vi "StirSticks.vi"(11 "RelayValue":T1) -> ()   [LabVIEW 2016]
uses:
  <vilib>/Rock Robotics/WPI/Relay/WPI_RelayValue.ctl
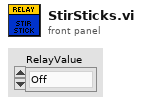
[diagram p1: front panel]
types:
  T1 = typedef "WPI_RelayValue.ctl" = enum16{"Off", "On", "Forward", "Reverse"}
  T2 = typedef "WPI_RelayDevRef.ctl" = cluster{"DevStatus":errorcluster, "Relay Channel":T3, "Relay Direction":T4}
  T3 = typedef "FPGA_DIORelayChannel.ctl" = enum8{"Relay 0", "Relay 1", "Relay 2", "Relay 3", "Invalid"}
  T4 = typedef "WPI_RelayDirection.ctl" = enum16{"Both directions", "Forward only", "Reverse only"}
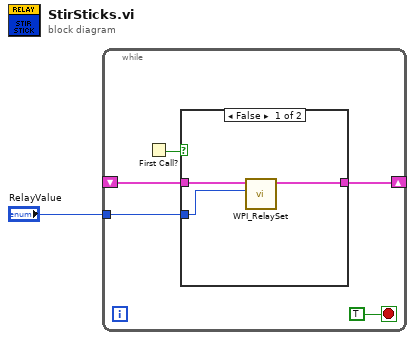
[diagram p0: block diagram]
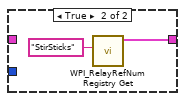
[diagram p2: hidden frame]
diagram:
  n1 = while {
    shift-right: [w4] -> _
    shift-left: _ -> [w3]
    tunnel: "RelayValue" -> [w2]
    stop <- TRUE stop-if-true
    n2 = First Call?() -> (First Call?: T/F=w5:bool)
    n3 = case shown="False" w5 {
      tunnel: [w8 w10] -> w4
      tunnel: w3 -> [w9 _]
      tunnel: w2 -> [w7 _]
      frame False {
        n4 = call <vilib>:"WPI_RelaySet.vi"("RelayValue"=w7, "RelayDevRef"=w9) -> ("RelayDevRef"=w8:T2)  [unwired: 8 in, 1 out]
      }
      frame True {
        n5 = call <vilib>:"WPI_RelayRefNum Registry Get.vi"("refnum name"="StirSticks") -> ("RelayDevRef"=w10:T2)  [unwired: 9 in, 1 out]
      }
    }
  }
